vi "Get Keithley meter Data.vi"(6 "INIT after?":bool=TRUE, 8 "error in (no error)":errorcluster, 10 "data string in":string=":FETCH?", 11 "VISA Resource Name":refnum<visa-resource-name>="GPIB0::20::INSTR") -> (0 "error out":errorcluster, 2 "Data":dbl format="%#_6p", 3 "VISA Resource Name Out":refnum<visa-resource-name>="GPIB0::20::INSTR")   [LabVIEW 2021]
uses:
  GPIB/VISA  Send Receive.vi
  Simple VISA Reader/Simple VISA Reader Driver.lvclass
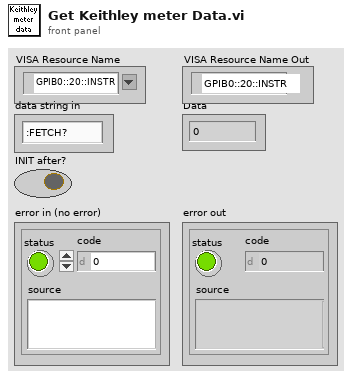
[diagram p1: front panel]
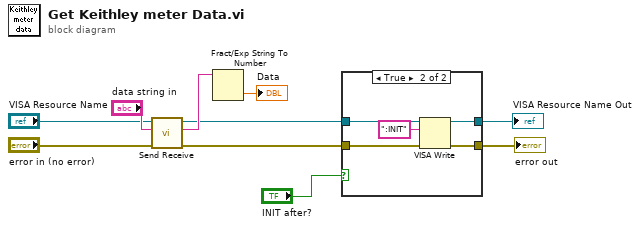
[diagram p0: block diagram]
diagram:
  n1 = call-poly "Send Receive.vi"("error in (no error)"="error in (no error)", "data string in"="data string in", "VISA Resource Name"="VISA Resource Name") -> ("error out"=w4:errorcluster, "data string out"=w8:string, "VISA Resource Name Out"=w6:refnum<visa-resource-name>)  [unwired: 6 in]
  n2 = Fract/Exp String To Number(string=w8) -> (number=→"Data":dbl)  [unwired: 4 out]
  n3 = case shown="True" "INIT after?" {
    tunnel: w6 -> [w11 w17]
    tunnel: [w11 w16] -> w5
    tunnel: w4 -> [w12 w15]
    tunnel: [w12 w14] -> w3
    frame False {
    }
    frame True {
      n4 = VISA Write(VISA resource name=w17, write buffer=":INIT", error in (no error)=w15) -> (VISA resource name out=w16:refnum<visa-resource-name>, error out=w14:errorcluster)  [unwired: 1 out]
    }
  }
  "error out" <- w3
  "VISA Resource Name Out" <- w5
